vi "RelayToggle.vi"(8 "error in":errorcluster, 10 "Power":bool, 11 "Relay":T1) -> (0 "error out":errorcluster)   [LabVIEW 2014]
uses:
  Type Defs/Relays.ctl
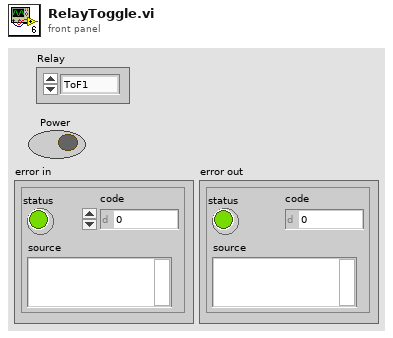
[diagram p1: front panel]
types:
  T1 = typedef "Relays.ctl" = enum16{"ToF1", "ToF2", "ToF3", "ToF4", "ToF5", "ToF6", "ToF7", "ToF8", "SensePwr", "All"}
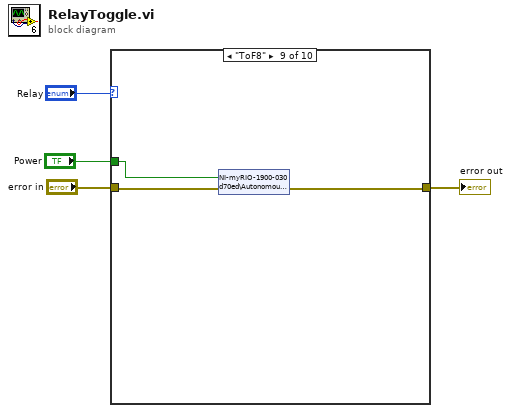
[diagram p0: block diagram]
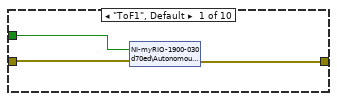
[diagram p2: hidden frame]
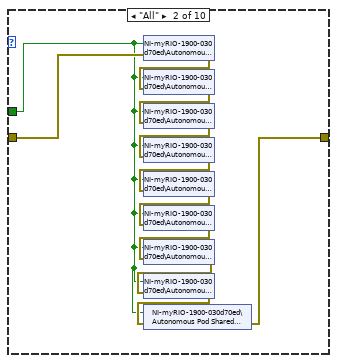
[diagram p3: hidden frame]
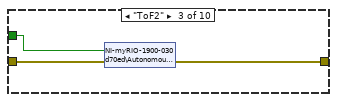
[diagram p4: hidden frame]
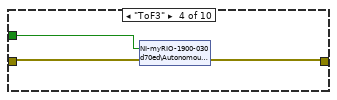
[diagram p5: hidden frame]
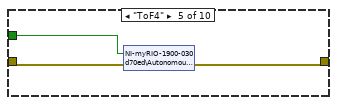
[diagram p6: hidden frame]
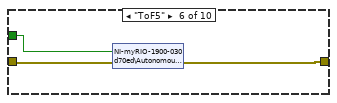
[diagram p7: hidden frame]
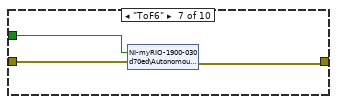
[diagram p8: hidden frame]
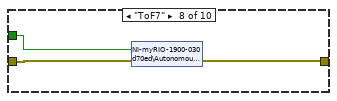
[diagram p9: hidden frame]
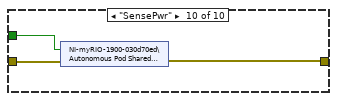
[diagram p10: hidden frame]
diagram:
  n1 = case shown="\"ToF8\"" "Relay" {
    tunnel: [w5 w10 w19 w22 w25 w28 w31 w34 w37 w41] -> w2
    tunnel: "error in" -> [w6 w9 w21 w24 w27 w30 w33 w36 w39 w42]
    tunnel: "Power" -> [w7 w8 w20 w23 w26 w29 w32 w35 w38 w40]
    frame "ToF1", Default {
      n2 = shared-variable "NI-myRIO-1900-030d70ed\\Autonomous Pod Shared Variables.lvlib\\ToF1"(w7, error in=w6) -> (error out=w5:errorcluster)
    }
    frame "All" {
      n3 = shared-variable "NI-myRIO-1900-030d70ed\\Autonomous Pod Shared Variables.lvlib\\ToF1"(w8, error in=w9) -> (error out=w11:errorcluster)
      n4 = shared-variable "NI-myRIO-1900-030d70ed\\Autonomous Pod Shared Variables.lvlib\\ToF2"(w8, error in=w11) -> (error out=w12:errorcluster)
      n5 = shared-variable "NI-myRIO-1900-030d70ed\\Autonomous Pod Shared Variables.lvlib\\ToF3"(w8, error in=w12) -> (error out=w13:errorcluster)
      n6 = shared-variable "NI-myRIO-1900-030d70ed\\Autonomous Pod Shared Variables.lvlib\\ToF4"(w8, error in=w13) -> (error out=w14:errorcluster)
      n7 = shared-variable "NI-myRIO-1900-030d70ed\\Autonomous Pod Shared Variables.lvlib\\ToF5"(w8, error in=w14) -> (error out=w15:errorcluster)
      n8 = shared-variable "NI-myRIO-1900-030d70ed\\Autonomous Pod Shared Variables.lvlib\\ToF6"(w8, error in=w15) -> (error out=w16:errorcluster)
      n9 = shared-variable "NI-myRIO-1900-030d70ed\\Autonomous Pod Shared Variables.lvlib\\ToF7"(w8, error in=w16) -> (error out=w17:errorcluster)
      n10 = shared-variable "NI-myRIO-1900-030d70ed\\Autonomous Pod Shared Variables.lvlib\\ToF8"(w8, error in=w17) -> (error out=w18:errorcluster)
      n11 = shared-variable "NI-myRIO-1900-030d70ed\\Autonomous Pod Shared Variables.lvlib\\SensePower"(w8, error in=w18) -> (error out=w10:errorcluster)
    }
    frame "ToF2" {
      n12 = shared-variable "NI-myRIO-1900-030d70ed\\Autonomous Pod Shared Variables.lvlib\\ToF2"(w20, error in=w21) -> (error out=w19:errorcluster)
    }
    frame "ToF3" {
      n13 = shared-variable "NI-myRIO-1900-030d70ed\\Autonomous Pod Shared Variables.lvlib\\ToF3"(w23, error in=w24) -> (error out=w22:errorcluster)
    }
    frame "ToF4" {
      n14 = shared-variable "NI-myRIO-1900-030d70ed\\Autonomous Pod Shared Variables.lvlib\\ToF4"(w26, error in=w27) -> (error out=w25:errorcluster)
    }
    frame "ToF5" {
      n15 = shared-variable "NI-myRIO-1900-030d70ed\\Autonomous Pod Shared Variables.lvlib\\ToF5"(w29, error in=w30) -> (error out=w28:errorcluster)
    }
    frame "ToF6" {
      n16 = shared-variable "NI-myRIO-1900-030d70ed\\Autonomous Pod Shared Variables.lvlib\\ToF6"(w32, error in=w33) -> (error out=w31:errorcluster)
    }
    frame "ToF7" {
      n17 = shared-variable "NI-myRIO-1900-030d70ed\\Autonomous Pod Shared Variables.lvlib\\ToF7"(w35, error in=w36) -> (error out=w34:errorcluster)
    }
    frame "ToF8" {
      n18 = shared-variable "NI-myRIO-1900-030d70ed\\Autonomous Pod Shared Variables.lvlib\\ToF8"(w38, error in=w39) -> (error out=w37:errorcluster)
    }
    frame "SensePwr" {
      n19 = shared-variable "NI-myRIO-1900-030d70ed\\Autonomous Pod Shared Variables.lvlib\\SensePower"(w40, error in=w42) -> (error out=w41:errorcluster)
    }
  }
  "error out" <- w2
